vi "Tracking v2.vi"(4 "Robot In":i32, 5 "Trajectory Cluster":T3, 6 "PID Cluster":T6={"L1 to L4 PID Cluster"={"L1 PID Gains"={"Kp"=0.005, "Kd"=0.5, "Ki"=0.0005}, "L2 PID Gains"={"Kp"=0.01, "Kd"=1.0, "Ki"=0.005}, "L3 PID Gains"={"Kp"=0.05, "Kd"=1.0, "Ki"=0.0005}, "L4 PID Gains"={"Kp"=0.1, "Kd"=0.1, "Ki"=0.0005}}, "Stage PID Cluster"={"Stage Z PID"={"Kp"=0.0005, "Kd"=0.001, "Ki"=0.0}, "Stage Y PID"={"Kp"=0.0003, "Kd"=0.01, "Ki"=0.0}, "Stage X PID"={"Kp"=0.0003, "Kd"=0.01, "Ki"=0.0}}, "OCT Z PID Gains"={"Kp"=0.0003, "Kd"=0.0001, "Ki"=0.01}}, 7 "Eye Model Cluster":T2={"X Grid"=[], "Y Grid"=[], "Za_true Surf"=[], "Iris Center"=[], "Zp_true Surf"=[], "Pinv"=[[1.0, 0.0], [0.0, 1.0]], "za_true"=5.0, "za_work"=1.0, "zp_work"=-1.0, "zp_true"=-5.0}, 8 "error in":errorcluster, 9 "Resume Index":i32, 10 "Prev Posit Cluster":T5={"Prev L1 to L4 Posit"=[-0.5319, -0.035669172703475985, -2.0566170657346783, 0.9099264705882353], "Prev Stage Posit"=[6.002553885707208, 5.996566124542428, 5.995469940427586], "Prev OCT Z Posit"=-0.0}, 11 "FPGA VI Reference In":refnum<k20>) -> (0 "error out":errorcluster, 1 "Leave Index":i32, 2 "Last Posit Cluster":T4={"Last L1 to L4 Posit"=[0.0, 0.0, 0.0, 0.0], "Last Stage Posit"=[6.0, 6.0, 6.0], "Last OCT Z Posit"=0.0}, 3 "FPGA VI Reference Out":refnum<k20>)   [LabVIEW 2016]
uses:
  Subsystems/Global Variables.vi
  <vilib>/Platform/TimedLoop/XDataNode/wakeup.ctl
  <vilib>/Platform/TimedLoop/XDataNode/XDNodeRunTimeDep.lvlib
  <vilib>/Platform/TimedLoop/XDataNode/nitl_modes.ctl
  <vilib>/Platform/TimedLoop/XDataNode/timing_clust.ctl
  <vilib>/platform/TimedLoop/XDataNode/XDataNode.xnode
  Library/KevinLibraryAll/labview/KevLib01.lvlib
  <vilib>/Utility/file.llb/Write Delimited Spreadsheet (string).vi
  <vilib>/Utility/file.llb/Write Delimited Spreadsheet (DBL).vi
  <vilib>/Analysis/Matrix/Datatypes/RealMatrix.ctl
  <vilib>/Analysis/Matrix/NI_Matrix.lvlib
panel:
  out "PC z Displacement":dbl
  out "Speed Schedule":dbl
  out "In Servo Loop":bool
  out "joint limits":dbl[][](array[numeric])=[[-10.0, 35.0], [-35.0, 35.0], [0.1, 10.0], [-40.0, 40.0]]
  out "Vac Extremum":dbl[](array[numeric])
  out "z Dist Thld":dbl[](array[numeric])
  out "z Rot Axis":dbl
  out "Deform Array":dbl[](array[numeric])=[1.0, 1.0, 1.0, 0.0, 0.0, 0.0, 0.0, 0.0, 0.0]
  out "Speed Override":u16(ring)=3 items=["4x", "3x", "2x", "1x", "0.5x", "0.2x", "0.1x", "PAUSE"]
  out "Loading Finished":bool
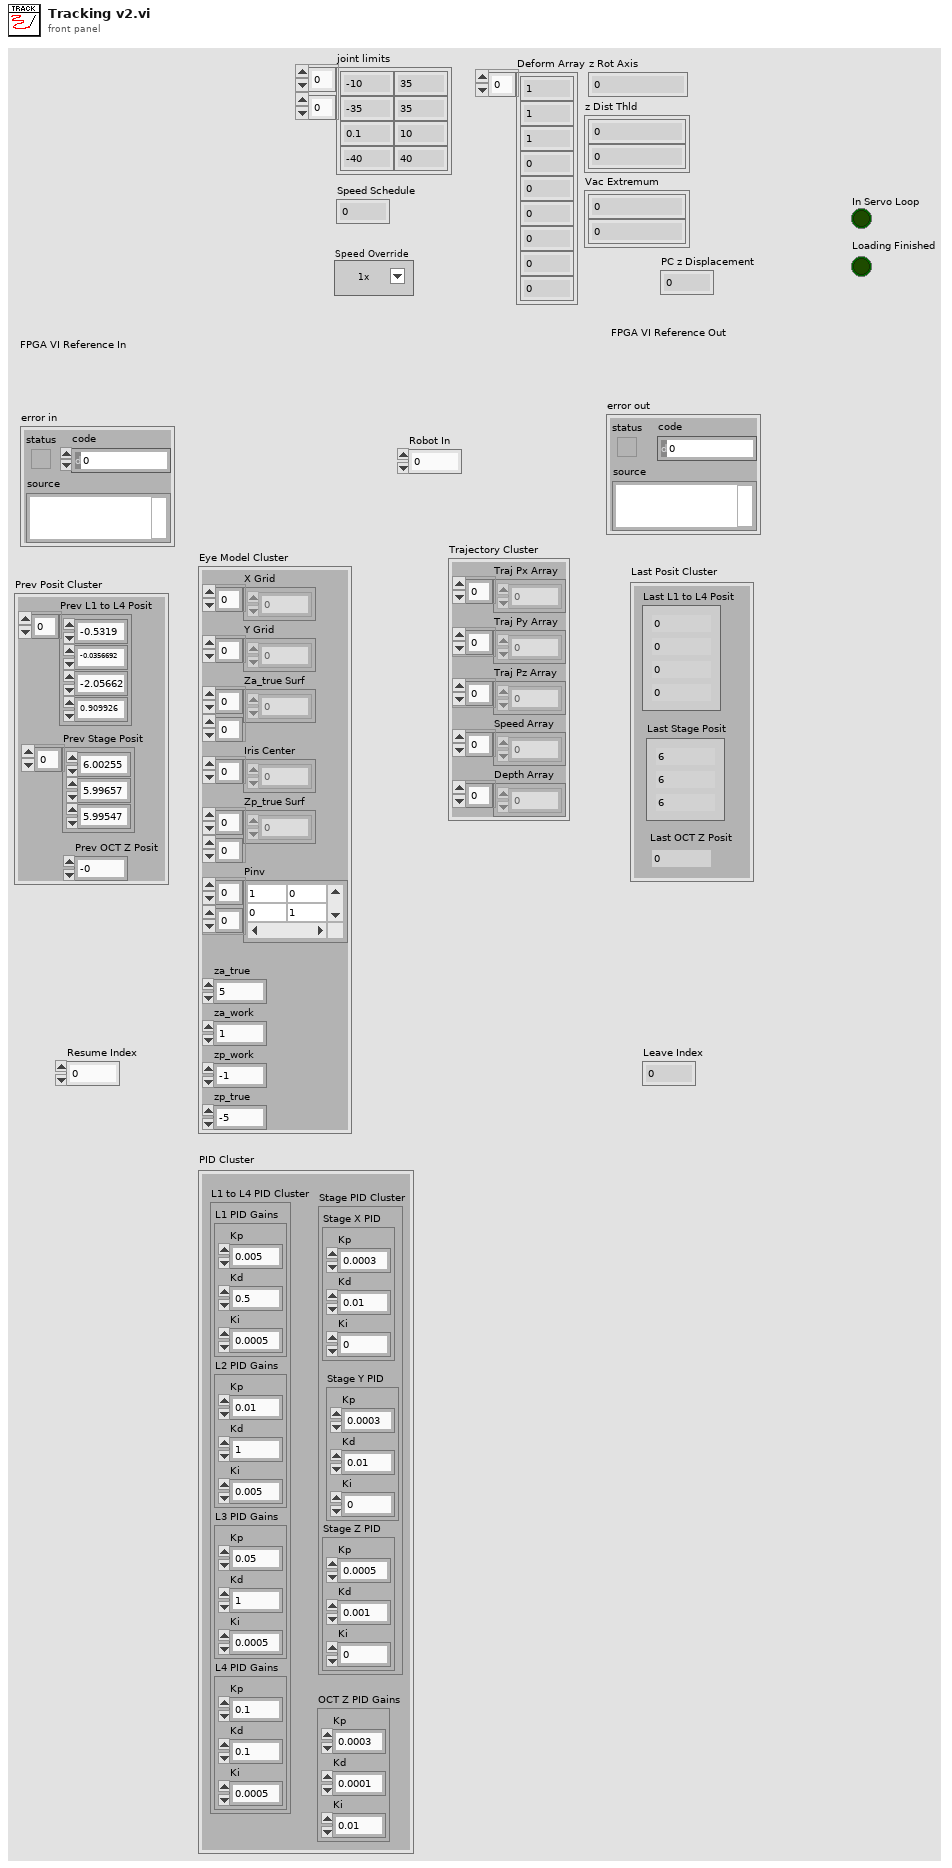
[diagram p1: front panel]
types:
  T1 = typedef "NI_Matrix.lvlib/RealMatrix.ctl" = dbl[][]
  T2 = cluster{"X Grid":dbl[], "Y Grid":dbl[], "Za_true Surf":dbl[][], "Iris Center":dbl[], "Zp_true Surf":dbl[][], "Pinv":T1, "za_true":dbl, "za_work":dbl, "zp_work":dbl, "zp_true":dbl}
  T3 = cluster{"Traj Px Array":dbl[], "Traj Py Array":dbl[], "Traj Pz Array":dbl[], "Speed Array":dbl[], "Depth Array":dbl[]}
  T4 = cluster{"Last L1 to L4 Posit":dbl[], "Last Stage Posit":dbl[], "Last OCT Z Posit":dbl}
  T5 = cluster{"Prev L1 to L4 Posit":dbl[], "Prev Stage Posit":dbl[], "Prev OCT Z Posit":dbl}
  T6 = cluster{"L1 to L4 PID Cluster":cluster{"L1 PID Gains":cluster{"Kp":dbl, "Kd":dbl, "Ki":dbl}, "L2 PID Gains":cluster{"Kp":dbl, "Kd":dbl, "Ki":dbl}, "L3 PID Gains":cluster{"Kp":dbl, "Kd":dbl, "Ki":dbl}, "L4 PID Gains":cluster{"Kp":dbl, "Kd":dbl, "Ki":dbl}}, "Stage PID Cluster":cluster{"Stage Z PID":cluster{"Kp":dbl, "Kd":dbl, "Ki":dbl}, "Stage Y PID":cluster{"Kp":dbl, "Kd":dbl, "Ki":dbl}, "Stage X PID":cluster{"Kp":dbl, "Kd":dbl, "Ki":dbl}}, "OCT Z PID Gains":cluster{"Kp":dbl, "Kd":dbl, "Ki":dbl}}
  T7 = typedef "XDNodeRunTimeDep.lvlib/timing_clust.ctl" = cluster{"Expected End [f-1]":u64, "Actual End [f-1]":u64, "Finished Late? [f-1]":bool, "Expected End [i-1]":u64, "Actual End [i-1]":u64, "Finished Late? [i-1]":bool, "Expected Start [i]":u64, "Actual Start [i]":u64, "Expected Start [f]":u64, "Actual Start [f]":u64, "Source Name":string, "Structure Name":string, "Period":i64, "Deadline":i64, "Offset":i64, "Start":i64, "Priority":i32, "Timeout":i32, "Mode":T8, "Wakeup Reason":T9, "Error":errorcluster, "Source Type":string, "Secondary Source Type":string, "Global End Time":u64, "Global Start Time":u64, "Frame Duration":u64, "Iteration Duration":u64, "Assigned CPU":i32, "I/O Scan Engine Mode":u32}
  T8 = typedef "XDNodeRunTimeDep.lvlib/nitl_modes.ctl" = enum32{"No Change", "Process missed periods, maintain original phase", "Discard missed periods, maintain original phase", "Process missed periods, ignore original phase", "Discard missed periods, ignore original phase"}
  T9 = typedef "XDNodeRunTimeDep.lvlib/wakeup.ctl" = enum32{"Normal", "Aborted", "Asynchronous wakeup", "Timing source error", "Timed loop error", "Timeout"}
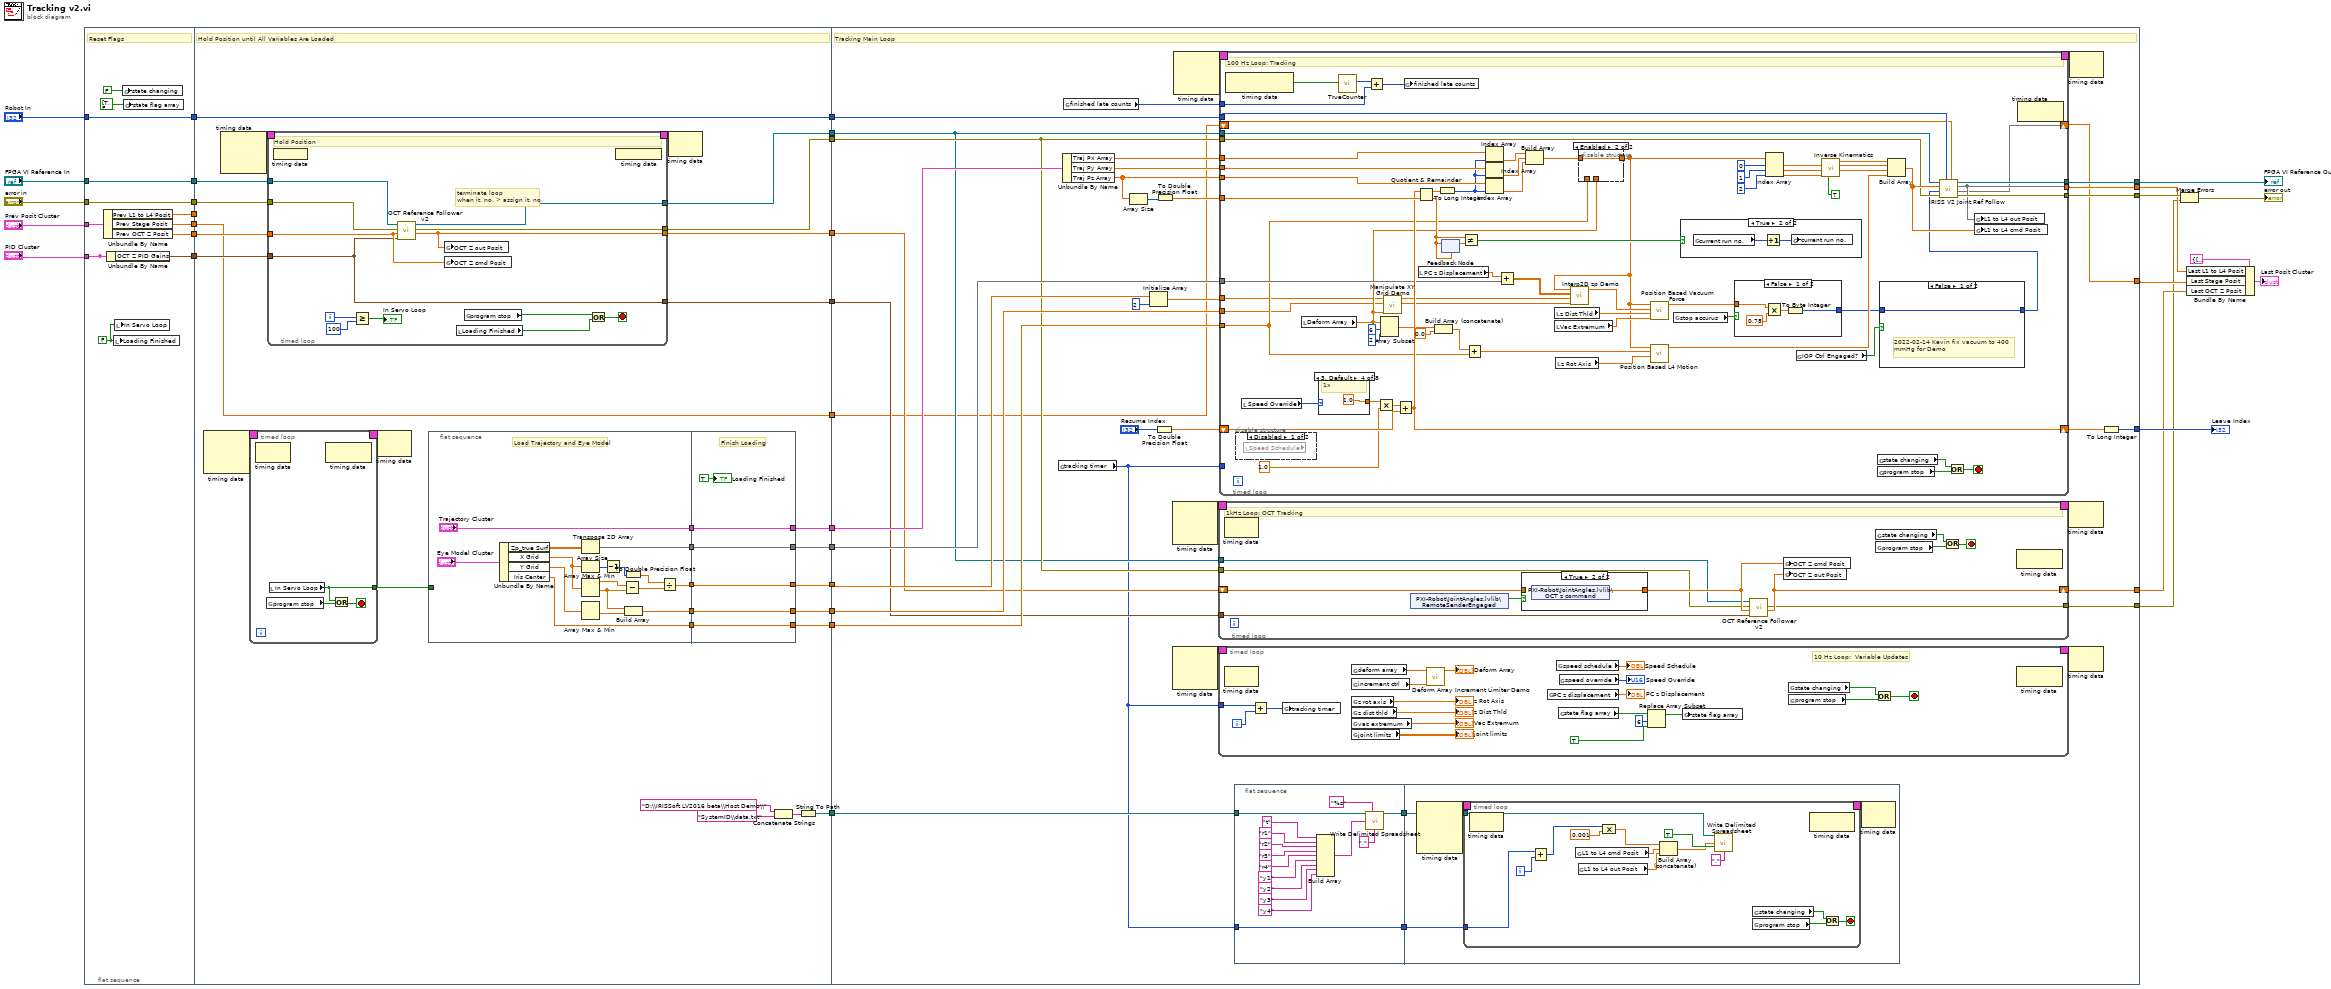
[diagram p0: block diagram]
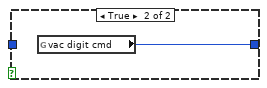
[diagram p4: hidden frame]
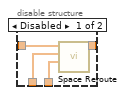
[diagram p5: hidden frame]
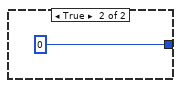
[diagram p6: hidden frame]
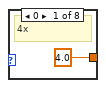
[diagram p7: hidden frame]
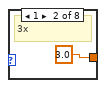
[diagram p8: hidden frame]
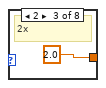
[diagram p9: hidden frame]
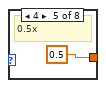
[diagram p10: hidden frame]
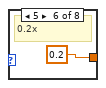
[diagram p11: hidden frame]
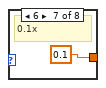
[diagram p12: hidden frame]
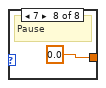
[diagram p13: hidden frame]
diagram:
  n1 = flat-sequence {
    tunnel: [w44] -> w34
    tunnel: "FPGA VI Reference In" -> [w44]
    tunnel: "error in" -> [w43]
    tunnel: [w43] -> w31
    tunnel: "Prev Posit Cluster" -> [w42]
    tunnel: [w41] -> _
    tunnel: "PID Cluster" -> [w41]
    tunnel: [w40] -> w28
    tunnel: [w39] -> w27
    tunnel: [w37] -> w14
    tunnel: [w36] -> w9
    tunnel: "Robot In" -> [w35]
    tunnel: [w35] -> w4
    tunnel: w34 -> [w75]
    tunnel: w31 -> [w74]
    tunnel: w28 -> [w51]
    tunnel: w27 -> [w73]
    tunnel: [w54] -> w26
    tunnel: [w72] -> w25
    tunnel: [w71] -> w17
    tunnel: [w70] -> w16
    tunnel: [w69] -> w15
    tunnel: w14 -> [_]
    tunnel: [w56] -> w13
    tunnel: [w63] -> w11
    tunnel: [w62] -> w10
    tunnel: w9 -> [w55]
    tunnel: [w53] -> w8
    tunnel: w4 -> [w53]
    tunnel: [w52] -> w3
    tunnel: [w51] -> w2
    tunnel: [w47] -> w1
    tunnel: w26 -> [w130]
    tunnel: w25 -> [w129]
    tunnel: [w157] -> w21
    tunnel: [w156] -> w20
    tunnel: [w155] -> w19
    tunnel: [w154] -> w18
    tunnel: w17 -> [w150]
    tunnel: w16 -> [w138]
    tunnel: w15 -> [w151]
    tunnel: w13 -> [w132]
    tunnel: [w146] -> w12
    tunnel: w11 -> [w139]
    tunnel: w10 -> [w140]
    tunnel: w8 -> [w135]
    tunnel: [w131] -> w7
    tunnel: [w128] -> w6
    tunnel: w3 -> [w127]
    tunnel: w2 -> [w126]
    tunnel: w1 -> [w125]
    frame #0 {
      w38 = FALSE ("Loading Finished")
      # "Reset Flags"
      n2 = Unbundle By Name(w42) -> ("Prev L1 to L4 Posit"=w37:dbl[], "Prev Stage Posit"=w40:dbl[], "Prev OCT Z Posit"=w39:dbl)
      n3 = Unbundle By Name(w41) -> ("OCT Z PID Gains"=w36:cluster{"Kp":dbl, "Kd":dbl, "Ki":dbl})
      n4 = local write "Loading Finished"(w38) -> ()
      n5 = local write "In Servo Loop"(w38) -> ()
      n6 = global write "Global Variables.vi" "state changing"(FALSE ("state changing")) -> ()
      n7 = global write "Global Variables.vi" "state flag array"(bool[] [TRUE, FALSE, FALSE, FALSE, FALSE, FALSE, FALSE, FALSE, FALSE] ("state flag array")) -> ()
    }
    frame #1 {
      # "terminate loop\nwhen it. no. > assign it. no."
      # "Hold Position until All Variables Are Loaded"
      n8 = node-c288() -> (w66:T7)  [unwired: 3 in]
      n9 = node-c288() -> (w68:T7)  [unwired: 3 in]
      n10 = timed-loop {
        timing: w66 -> [_]
        timing-out: [_] -> w65
        tunnel: [w98] -> w64
        stop <- w100 stop-if-true
        n11 = node-c288() -> ()  [unwired: 1 in, 1 out]
        n12 = global read "Global Variables.vi" "program stop"() -> (w99:bool)
        n13 = local read "In Servo Loop"() -> (w98:bool)
        n14 = node-c288() -> ()  [unwired: 1 in, 1 out]
        n15 = Or(x=w98, y=w99) -> (x .or. y?=w100:bool)
      }
      n16 = timed-loop {
        timing: w68 -> [_]
        timing-out: [_] -> w67
        tunnel: [w108] -> w56
        tunnel: [w105] -> w52
        tunnel: [w109] -> w54
        tunnel: w75 -> [w111]
        tunnel: w74 -> [w110]
        tunnel: w55 -> [w106]
        tunnel: w73 -> [w107]
        tunnel: [w106] -> w72
        i -> [w114]
        stop <- w117 stop-if-true
        # "Hold Position"
        n17 = node-c288 ("Output Node")() -> ()  [unwired: 1 in]
        n18 = Greater Or Equal?(x=w114, y=100) -> (x >= y?=→"In Servo Loop":bool)
        n19 = call "OCT Reference Follower v2.vi"("OCT Z PID Gains"=w106, "OCT  Z cmd Posit [mm]"=w107, "error in"=w110, "FPGA VI Reference In"=w111) -> ("OCT  Z out Posit [mm]"=w108:dbl, "error out"=w109:errorcluster, "FPGA VI Reference Out"=w105:refnum<k20>)  [unwired: 5 in]
        n20 = global write "Global Variables.vi" "OCT Z out Posit"(w108) -> ()
        n21 = global write "Global Variables.vi" "OCT Z cmd Posit"(w107) -> ()
        n22 = local read "Loading Finished"() -> (w116:bool)
        n23 = global read "Global Variables.vi" "program stop"() -> (w115:bool)
        n24 = Or(x=w115, y=w116) -> (x .or. y?=w117:bool)
        n25 = node-c288() -> ()  [unwired: 1 out]
      }
      n26 = node-c288(w65) -> ()  [unwired: 1 out]
      n27 = flat-sequence {
        tunnel: [w78] -> w61
        tunnel: [w91] -> w60
        tunnel: [w90] -> w59
        tunnel: [w77] -> w58
        tunnel: ["Trajectory Cluster"] -> w57
        tunnel: w64 -> [_]
        tunnel: [w95] -> w69
        tunnel: [w96] -> w70
        tunnel: [w97] -> w71
        tunnel: w61 -> [w97]
        tunnel: w60 -> [w96]
        tunnel: w59 -> [w95]
        tunnel: w58 -> [w93]
        tunnel: [w93] -> w63
        tunnel: [w92] -> w62
        tunnel: w57 -> [w92]
        frame #0 {
          # "Load Trajectory and Eye Model"
          n28 = Unbundle By Name("Eye Model Cluster") -> ("Zp_true Surf"=w79:dbl[][], "X Grid"=w80:dbl[], "Y Grid"=w89:dbl[], "Iris Center"=w77:dbl[])
          n29 = Transpose 2D Array(2D array=w79) -> (transposed array=w78:dbl[][])
          n30 = Array Size(array=w80) -> (size(s)=w88:i32)
          n31 = Array Max & Min(array=w80) -> (max value=w86:dbl, min value=w87:dbl)  [unwired: 2 out]
          n32 = Array Max & Min(array=w89) -> (min value=w85:dbl)  [unwired: 3 out]
          n33 = Decrement(x=w88) -> (x-1=w83:i32)
          n34 = Subtract(x=w86, y=w87) -> (x-y=w82:dbl)
          n35 = To Double Precision Float(number=w83) -> (double precision float=w84:dbl)
          n36 = Build Array(w87, w85) -> (w90:dbl[])
          n37 = Divide(x=w84, y=w82) -> (x/y=w91:dbl)
        }
        frame #1 {
          # "Finish Loading"
          "Loading Finished" <- TRUE ("Loading Finished")
        }
      }
      n38 = node-c288(w67) -> ()  [unwired: 1 out]
      n39 = Concatenate Strings("D:\\IRISSoft LV2016 beta\\Host Demo\\", "SystemID\\data.txt") -> (w50:string)
      n40 = String To Path(string=w50) -> (path=w47:path)
    }
    frame #2 {
      # "Tracking Main Loop"
      n41 = global read "Global Variables.vi" "tracking timer"() -> (w124:i32)
      n42 = Unbundle By Name(w140) -> ("Traj Px Array"=w149:dbl[], "Traj Py Array"=w148:dbl[], "Traj Pz Array"=w143:dbl[])
      n43 = global read "Global Variables.vi" "finished late counts"() -> (w158:u16)
      n44 = Array Size(array=w143) -> (size(s)=w142:i32)
      n45 = Initialize Array(w138, 2 ("dimension size")) -> (w136:dbl[])
      n46 = To Double Precision Float(number="Resume Index") -> (double precision float=w145:dbl)
      n47 = To Double Precision Float(number=w142) -> (double precision float=w141:dbl)
      n48 = node-c288() -> (w134:T7)  [unwired: 3 in]
      n49 = node-c288() -> (w153:T7)  [unwired: 3 in]
      n50 = node-c288() -> (w160:T7)  [unwired: 3 in]
      n51 = timed-loop {
        timing: w134 -> [_]
        timing-out: [_] -> w133
        shift-right: [w203] -> w131
        shift-left: w132 -> [w204]
        tunnel: w127 -> [w202]
        tunnel: w130 -> [w201]
        tunnel: w129 -> [w200]
        tunnel: [w199] -> w128
        stop <- w208 stop-if-true
        # "1kHz Loop: OCT Tracking"
        n52 = node-c288() -> ()  [unwired: 1 in, 1 out]
        n53 = shared-variable "PXI-Robot\\JointAngles.lvlib\\RemoteSenderEngaged"() -> (w198:bool)  [unwired: 1 in, 1 out]
        n54 = case shown="True" w198 {
          tunnel: [w209 w210] -> w205
          tunnel: w204 -> [w209 _]
          frame False {
            # "Hold Position if not Engaged"
          }
          frame True {
            n55 = shared-variable "PXI-Robot\\JointAngles.lvlib\\OCT z command"() -> (w210:dbl)  [unwired: 1 in, 1 out]
          }
        }
        n56 = call "OCT Reference Follower v2.vi"("OCT Z PID Gains"=w200, "OCT  Z cmd Posit [mm]"=w205, "error in"=w201, "FPGA VI Reference In"=w202) -> ("OCT  Z out Posit [mm]"=w203:dbl, "error out"=w199:errorcluster)  [unwired: 5 in, 1 out]
        n57 = global write "Global Variables.vi" "OCT Z cmd Posit"(w205) -> ()
        n58 = global write "Global Variables.vi" "OCT Z out Posit"(w203) -> ()
        n59 = global read "Global Variables.vi" "state changing"() -> (w207:bool)
        n60 = global read "Global Variables.vi" "program stop"() -> (w206:bool)
        n61 = Or(x=w207, y=w206) -> (x .or. y?=w208:bool)
        n62 = node-c288() -> ()  [unwired: 1 in, 1 out]
      }
      n63 = timed-loop {
        timing: w153 -> [_]
        timing-out: [_] -> w152
        tunnel: w124 -> [w218]
        i -> [w219]
        stop <- w234 stop-if-true
        # "10 Hz Loop:  Variable Updates"
        n64 = node-c288() -> ()  [unwired: 1 in, 1 out]
        n65 = Add(x=w218, y=w219) -> (x+y=w220:i32)
        n66 = global write "Global Variables.vi" "tracking timer"(w220) -> ()
        n67 = global read "Global Variables.vi" "deform array"() -> (w217:dbl[])
        n68 = global read "Global Variables.vi" "increment ctrl"() -> (w216:dbl[])
        n69 = global read "Global Variables.vi" "z rot axis"() -> (→"z Rot Axis":dbl)
        n70 = global read "Global Variables.vi" "z dist thld"() -> (→"z Dist Thld":dbl[])
        n71 = global read "Global Variables.vi" "vac extremum"() -> (→"Vac Extremum":dbl[])
        n72 = global read "Global Variables.vi" "joint limits"() -> (→"joint limits":dbl[][])
        n73 = call "Deform Array Increment Limiter Demo.vi"("Increment Array"=w216, "Defrom Ref"=w217) -> ("Deform Output"=→"Deform Array":dbl[])  [unwired: 9 in]
        n74 = global read "Global Variables.vi" "PC z displacement"() -> (→"PC z Displacement":dbl)
        n75 = global read "Global Variables.vi" "speed schedule"() -> (→"Speed Schedule":dbl)
        n76 = global read "Global Variables.vi" "state flag array"() -> (w223:bool[])
        n77 = global read "Global Variables.vi" "speed override"() -> (→"Speed Override":u16)
        n78 = Replace Array Subset(array=w223, new element=TRUE ("new element/subarray"), index=6) -> (w224:bool[])
        n79 = global write "Global Variables.vi" "state flag array"(w224) -> ()
        n80 = global read "Global Variables.vi" "state changing"() -> (w233:bool)
        n81 = global read "Global Variables.vi" "program stop"() -> (w232:bool)
        n82 = Or(x=w233, y=w232) -> (x .or. y?=w234:bool)
        n83 = node-c288() -> ()  [unwired: 1 in, 1 out]
      }
      n84 = timed-loop {
        timing: w160 -> [_]
        timing-out: [_] -> w159
        tunnel: w149 -> [w309]
        tunnel: w148 -> [w308]
        tunnel: w143 -> [w300]
        tunnel: w127 -> [w268]
        tunnel: w130 -> [w266]
        tunnel: [w265] -> w157
        tunnel: w158 -> [w302]
        shift-right: [w240] -> w154
        shift-left: w126 -> [w239]
        tunnel: [w264] -> w156
        tunnel: [w246] -> w155
        shift-right: [w287] -> w147
        shift-left: w145 -> [w290]
        tunnel: w150 -> [w283]
        tunnel: w136 -> [w280]
        tunnel: w151 -> [w279]
        tunnel: w141 -> [w289]
        tunnel: w139 -> [w282]
        tunnel: w124 -> [_]
        tunnel: w135 -> [w269]
        stop <- w306 stop-if-true
        # "100 Hz Loop: Tracking"
        n85 = node-c288() -> (w305:bool)  [unwired: 1 in]
        n86 = disable-structure shown="Disabled" {
          frame Disabled {
            n87 = local read "Speed Schedule"() -> ()  [unwired: 1 out]
          }
          frame Enabled {
          }
        }
        n88 = local read "Speed Override"() -> (w292:u16)
        n89 = local read "Deform Array"() -> (w281:dbl[])
        n90 = case shown="3, Default" w292 {
          tunnel: [4.0 ("y") 3.0 ("y") 2.0 ("y") 1.0 ("y") 0.5 ("y") 0.2 ("y") 0.1 ("y") 0.0 ("y")] -> w291
          frame 0 {
            # "4x"
          }
          frame 1 {
            # "3x"
          }
          frame 2 {
            # "2x"
          }
          frame 3, Default {
            # "1x"
          }
          frame 4 {
            # "0.5x"
          }
          frame 5 {
            # "0.2x"
          }
          frame 6 {
            # "0.1x"
          }
          frame 7 {
            # "Pause"
          }
        }
        n91 = call "TrueCounter.vi"("True?"=w305) -> ("True Count"=w303:u16)  [unwired: 10 in]
        n92 = Add(x=w303, y=w302) -> (x+y=w304:u16)
        n93 = Multiply(x=w291, y=1.0) -> (x*y=w293:dbl)
        n94 = Array Subset(array=w281, index=6, length=2) -> (w259:dbl[])
        n95 = call "Manipulate XY Grid Demo.vi"("Deform Array"=w281, "XY Grid min In"=w279, "XY Quant. Fact. In"=w280) -> ("XY Grid min Out"=w254:dbl[], "XY Quant. Fact. Out"=w255:dbl[])  [unwired: 7 in]
        n96 = Add(x=w293, y=w290) -> (x+y=w287:dbl)
        n97 = global write "Global Variables.vi" "finished late counts"(w304) -> ()
        n98 = Quotient & Remainder(x=w287, y=w289) -> (x-y*floor(x/y)=w288:dbl, floor(x/y)=w284:dbl)
        n99 = local read "PC z Displacement"() -> (w262:dbl)
        n100 = Build Array (concatenate)(w259, 0.0) -> (w258:dbl[])
        n101 = To Long Integer(number=w288) -> (32bit integer=w245:i32)
        n102 = feedback-in #1(w284) -> ()
        n103 = feedback #1(w284) -> (w286:dbl)
        n104 = Not Equal?(x=w284, y=w286) -> (x != y?=w285:bool)
        n105 = Add(x=w258, y=w282) -> (x+y=w249:dbl[])
        n106 = Index Array(array=w309, index=w245) -> (element=w296:dbl)
        n107 = Index Array(array=w308, index=w245) -> (element=w295:dbl)
        n108 = Index Array(array=w300, index=w245) -> (element=w294:dbl)
        n109 = Add(x=w262, y=w283) -> (x+y=w256:dbl[][])
        n110 = Build Array(w296, w295, w294) -> (w277:dbl[])
        n111 = local read "z Dist Thld"() -> (w252:dbl[])
        n112 = local read "Vac Extremum"() -> (w251:dbl[])
        n113 = local read "z Rot Axis"() -> (w248:dbl)
        n114 = disable-structure shown="Enabled" {
          disable-tunnel: w282 -> [w315 _]
          disable-tunnel: w281 -> [w314 _]
          disable-tunnel: w277 -> [w313 w316]
          disable-tunnel: [w312 w316] -> w247
          frame Disabled {
            n115 = call "Space Reroute.vi"("Deform Array"=w314, "Pivot Pt"=w315, "Nominal Traj Pt"=w313) -> ("Reroute Traj Pt"=w312:dbl[])  [unwired: 8 in]
          }
          frame Enabled {
          }
        }
        n116 = call "Interp2D zp Demo.vi"("XY Grid min"=w254, "XY Quantization Factor"=w255, "Zp array"=w256, "Tip Position"=w247) -> ("zp"=w253:dbl)  [unwired: 7 in]
        n117 = call "Position Based Vacuum Force.vi"("vac_bnd"=w251, "z_thld"=w252, "current zp"=w253, "tip position"=w247) -> ("vacf (%)"=w250:dbl)  [unwired: 7 in]
        n118 = call "Position Based L4 Motion.vi"("Assign z"=w248, "Iris Center"=w249, "Tip Position"=w247) -> ("L4 Motion [deg]"=w278:dbl)  [unwired: 8 in]
        n119 = global read "Global Variables.vi" "stop accurus"() -> (w263:bool)
        n120 = case shown="True" w285 {
          frame False {
          }
          frame True {
            n121 = global read "Global Variables.vi" "current run no."() -> (w331:u8)
            n122 = Increment(x=w331) -> (x+1=w330:u8)
            n123 = global write "Global Variables.vi" "current run no."(w330) -> ()
          }
        }
        n124 = case shown="False" w263 {
          tunnel: w250 -> [w318 _]
          tunnel: [w317 i8 0 ("Digital Cmd [0-78]")] -> w242
          frame False {
            n125 = Multiply(x=w318, y=0.78 ("x")) -> (x*y=w319:dbl)
            n126 = To Byte Integer(number=w319) -> (8bit integer=w317:i8)
          }
          frame True {
          }
        }
        n127 = Index Array(array=w247, index #1=0 ("index"), index #2=1 ("index"), index #3=2 ("index")) -> (element #1=w275:dbl, element #2=w274:dbl, element #3=w273:dbl)
        n128 = global read "Global Variables.vi" "IOP Ctrl Engaged?"() -> (w244:bool)
        n129 = call "Inverse Kinematics.vi"("isToolTipInsideEye"=TRUE, "z"=w273, "y"=w274, "x"=w275) -> ("j3"=w270:dbl, "j2"=w271:dbl, "j1"=w272:dbl)  [unwired: 4 in, 1 out]
        n130 = global read "Global Variables.vi" "state changing"() -> (w301:bool)
        n131 = global read "Global Variables.vi" "program stop"() -> (w307:bool)
        n132 = case shown="False" w244 {
          tunnel: [w310 w311] -> w243
          tunnel: w242 -> [w310 _]
          frame False {
            # "2022-02-14 Kevin fix vacuum to 400 mmHg for Demo"
          }
          frame True {
            n133 = global read "Global Variables.vi" "vac digit cmd"() -> (w311:i8)
          }
        }
        n134 = Build Array(w272, w271, w270, w278) -> (w267:dbl[])
        n135 = call "IRISS V2 Joint Ref Follow.vi"(4:w239, 5:w269, "error in"=w266, "Digital Cmd [0-78]"=w243, 8:w267, "FPGA VI Reference In"=w268) -> ("error out"=w264:errorcluster, 1:w240, 2:w246, "FPGA VI Reference Out"=w265:refnum<k20>)
        n136 = Or(x=w301, y=w307) -> (x .or. y?=w306:bool)
        n137 = global write "Global Variables.vi" "L1 to L4 out Posit"(w246) -> ()
        n138 = global write "Global Variables.vi" "L1 to L4 cmd Posit"(w267) -> ()
        n139 = node-c288() -> ()  [unwired: 1 in, 1 out]
      }
      n140 = flat-sequence {
        tunnel: [w163] -> w123
        tunnel: w125 -> [w162]
        tunnel: [w161] -> w122
        tunnel: w124 -> [w161]
        tunnel: w123 -> [w179]
        tunnel: w122 -> [w178]
        frame #0 {
          n141 = Build Array("t" ("delimiter (\\t)"), "r1" ("delimiter (\\t)"), "r2" ("delimiter (\\t)"), "r3" ("delimiter (\\t)"), "r4" ("delimiter (\\t)"), "y1" ("delimiter (\\t)"), "y2" ("delimiter (\\t)"), "y3" ("delimiter (\\t)"), "y4" ("delimiter (\\t)")) -> (w168:string[])
          n142 = call-poly <vilib>:"Write Delimited Spreadsheet.vi"("file path (dialog if empty)"=w162, "format (%s)"="%s", "1D data"=w168, "delimiter (\\t)"="," ("delimiter (\\t)")) -> ("new file path (Not A Path if cancelled)"=w163:path)  [unwired: 10 in, 1 out]
        }
        frame #1 {
          n143 = node-c288() -> (w177:T7)  [unwired: 4 in]
          n144 = timed-loop {
            tunnel: w179 -> [w189]
            tunnel: w178 -> [w183]
            timing: w177 -> [_]
            timing-out: [_] -> w176
            i -> [w182]
            stop <- w184 stop-if-true
            n145 = node-c288() -> ()  [unwired: 1 in, 1 out]
            n146 = Add(x=w183, y=w182) -> (x+y=w181:i32)
            n147 = global read "Global Variables.vi" "L1 to L4 cmd Posit"() -> (w191:dbl[])
            n148 = global read "Global Variables.vi" "L1 to L4 out Posit"() -> (w180:dbl[])
            n149 = Compound Arithmetic op=MULTIPLY(w181, 0.001 ("y")) -> (w187:dbl)
            n150 = Build Array (concatenate)(w187, w191, w180) -> (w190:dbl[])
            n151 = call-poly <vilib>:"Write Delimited Spreadsheet.vi"("file path (dialog if empty)"=w189, "1D data"=w190, "append to file? (new file:F)"=TRUE, "delimiter (\\t)"="," ("delimiter (\\t)")) -> ()  [unwired: 10 in, 2 out]
            n152 = global read "Global Variables.vi" "state changing"() -> (w186:bool)
            n153 = global read "Global Variables.vi" "program stop"() -> (w185:bool)
            n154 = node-c288() -> ()  [unwired: 1 in, 1 out]
            n155 = Or(x=w186, y=w185) -> (x .or. y?=w184:bool)
          }
          n156 = node-c288(w176) -> ()  [unwired: 1 out]
        }
      }
      n157 = node-c288(w133) -> ()  [unwired: 1 out]
      n158 = node-c288(w152) -> ()  [unwired: 1 out]
      n159 = node-c288(w159) -> ()  [unwired: 1 out]
      n160 = To Long Integer(number=w147) -> (32bit integer=w146:i32)
    }
  }
  n161 = Merge Errors(w20, w6) -> (→"error out":errorcluster)
  n162 = Bundle By Name(cluster=T4 {"Last L1 to L4 Posit"=[0.0, 0.0, 0.0, 0.0], "Last Stage Posit"=[6.0, 6.0, 6.0], "Last OCT Z Posit"=0.0} ("Last Posit Cluster 2"), "Last L1 to L4 Posit"=w19, "Last Stage Posit"=w18, "Last OCT Z Posit"=w7) -> (→"Last Posit Cluster":T4)
  "FPGA VI Reference Out" <- w21
  "Leave Index" <- w12
